vi "Target Distance.vi"(10 "Target":dbl[](array[numeric]), 11 "Position":dbl[](array[numeric])) -> (3 "Target Distance":dbl)   [LabVIEW 2016]
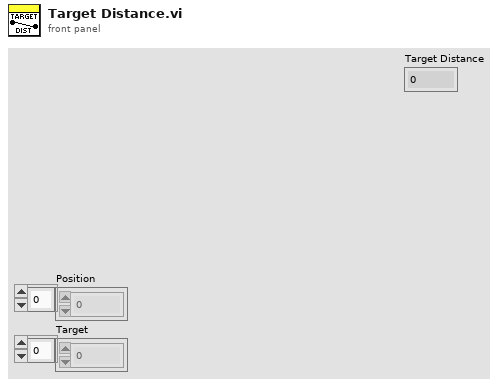
[diagram p1: front panel]
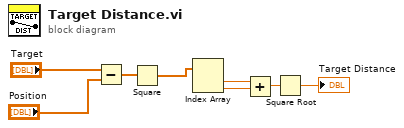
[diagram p0: block diagram]
diagram:
  n1 = Subtract(x="Target", y="Position") -> (x-y=w6:dbl[])
  n2 = Square(x=w6) -> (x^2=w5:dbl[])
  n3 = Index Array(array=w5) -> (element #1=w3:dbl, element #2=w4:dbl)  [unwired: 2 in]
  n4 = Add(x=w3, y=w4) -> (x+y=w2:dbl)
  n5 = Square Root(x=w2) -> (sqrt(x)=→"Target Distance":dbl)
